vi "CODMn启动 (子VI).vi"(11 "启动测量模式":T2) -> (0 "error out":T1={"status"=FALSE, "代码"=4, "source"=""} caption="错误输出" {"代码" items=["执行成功"=1, "执行失败，但不知道原因"=2, "命令请求条件错误"=3, "通讯超时"=4, "系统繁忙不能执行"=5, "系统故障"=6, "没有数据"=100]})   [LabVIEW 2016, in "MB SLAVE.lvlib"]
uses:
  MB SLAVE.lvlib
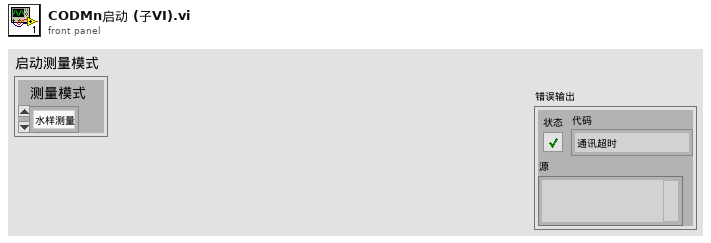
[diagram p1: front panel]
types:
  T1 = cluster{"status":bool, "代码":u16, "source":string}
  T2 = cluster{"测量模式":enum16{"水样测量", "标样核查", "零点核查", "跨度核查", "空白测试", "加标回收", "平行样", "校零", "校标"}}
  T3 = enum16{"空闲", "水样测试", "标样核查", "零点核查", "跨度核查", "空白测试", "平行样测试", "质控样", "空白校准", "标样校准", "加标回收"}
  T4 = typedef "CODMn交互.ctl" = cluster{"COD浓度（mg/L)":dbl, "水样启动时间":timestamp, "加标回收启动时间":timestamp, "CODMn工作状态":enum16{"空闲", "水样测试", "标样核查", "零点核查", "跨度核查", "空白测试", "平行样测试", "加标回收", "空白校准", "标样校准", "初始化（清洗）"}, "多列列表框":i32, "平台试剂余量百分比":sgl, "CODMn仪器参数":cluster{"测量量程":dbl, "测量精度":dbl, "测量间隔":dbl, "消解温度":dbl, "消解时长":dbl, "空白校准时间":timestamp, "曲线截距":dbl, "曲线斜率":dbl, "测量检出限":dbl, "测量信号值":dbl, "线性相关系数":dbl, "二次多项式系数":dbl, "标样校准时间":timestamp, "稀释倍数":dbl, "三项式系数":dbl, "空白标定系数":dbl, "量程系数":dbl, "F0/ORPA":dbl, "F1/ORPB":dbl, "F2/ORPK":dbl, "F3":dbl, "F4":dbl, "F5":dbl, "F6":dbl, "F7":dbl, "X0/滴定数":dbl, "量程":dbl}}
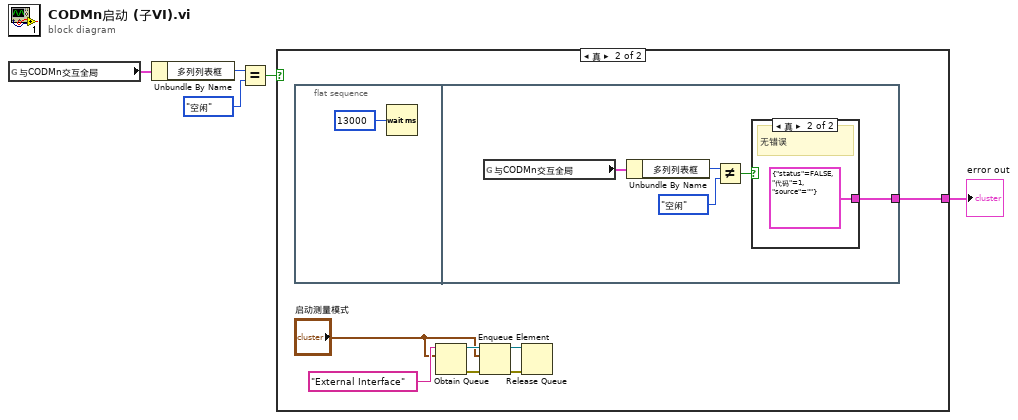
[diagram p0: block diagram]
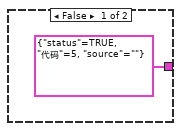
[diagram p2: hidden frame]
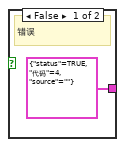
[diagram p3: hidden frame]
diagram:
  n1 = global read "modbus slave全局.vi" "与CODMn交互全局"() -> (w2:T4)
  n2 = Unbundle By Name(w2) -> ("多列列表框"=w1:i32)
  n3 = Equal?(x=w1, y=T3."空闲") -> (x = y?=w4:bool)
  n4 = case shown="真" w4 {
    tunnel: [T1 {"status"=TRUE, "代码"=5, "source"=""} ("error out") w13] -> w3
    frame False {
    }
    frame True {
      n5 = flat-sequence {
        tunnel: [w17] -> w13
        frame #0 {
          n6 = Wait (ms)(milliseconds to wait=u32 13000 ("等待时间（毫秒）")) -> ()  [unwired: 1 out]
        }
        frame #1 {
          n7 = global read "modbus slave全局.vi" "与CODMn交互全局"() -> (w16:T4)
          n8 = Unbundle By Name(w16) -> ("多列列表框"=w15:i32)
          n9 = Not Equal?(x=w15, y=T3."空闲") -> (x != y?=w18:bool)
          n10 = case shown="真" w18 {
            tunnel: [T1 {"status"=TRUE, "代码"=4, "source"=""} ("error out") T1 {"status"=FALSE, "代码"=1, "source"=""} ("error out")] -> w17
            frame False {
              # "错误"
            }
            frame True {
              # "无错误"
            }
          }
        }
      }
      n11 = Obtain Queue(name (unnamed)="External Interface" ("名称（未命名）"), element data type="启动测量模式") -> (queue out=w11:refnum<queue>, error out=w10:errorcluster)  [unwired: 3 in, 1 out]
      n12 = Enqueue Element(queue=w11, element="启动测量模式", error in (no error)=w10) -> (queue out=w9:refnum<queue>, error out=w8:errorcluster)  [unwired: 1 in, 1 out]
      n13 = Release Queue(queue=w9, error in (no error)=w8) -> ()  [unwired: 1 in, 3 out]
    }
  }
  "error out" <- w3
